vi "Cipher to Number.vi"(8 "error in (no error)":errorcluster, 11 "Cipers":i32[](array[numeric])) -> (0 "error out":errorcluster, 1 "Negative":bool, 3 "Number":i32)   [LabVIEW 2018, in "Resistance Values.lvlib"]
uses:
  Resistance Values.lvlib
  <vilib>/Utility/error.llb/Error Cluster From Error Code.vi
  <vilib>/ErrorRing/Error Ring.xnode
panel:
  # "index = 0 ->LDS"
  # "index = 1 ->......"
  # "index = n -> MDS"
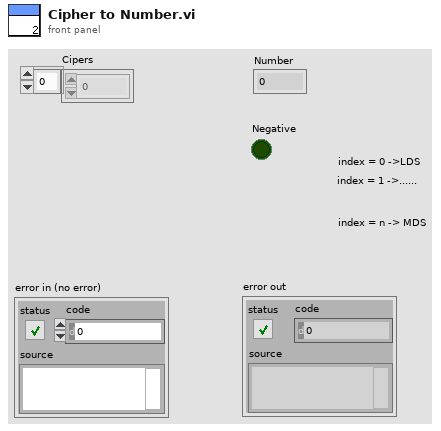
[diagram p1: front panel]
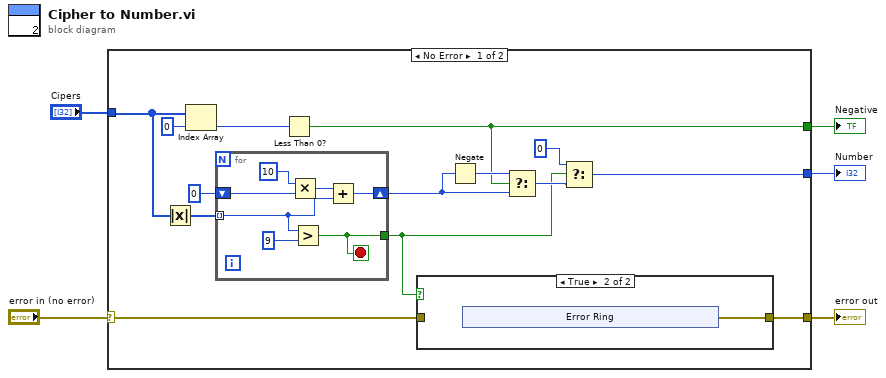
[diagram p0: block diagram]
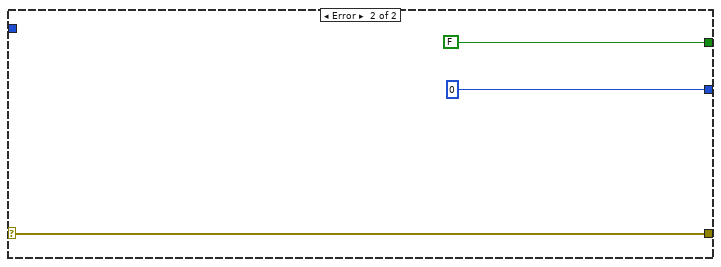
[diagram p3: hidden frame]
diagram:
  n1 = case shown="No Error" "error in (no error)" {
    selector: "error in (no error)" -> [w8 w36]
    tunnel: "Cipers" -> [w16 _]
    tunnel: [w13 FALSE] -> w3
    tunnel: [w9 0] -> w2
    tunnel: [w6 w36] -> w1
    frame No Error {
      n2 = Absolute Value(x=w16) -> (abs(x)=w17:i32[])
      n3 = Index Array(array=w16, index=0) -> (element=w18:i32)
      n4 = for {
        tunnel: w17 -> [w29] mode=indexing
        shift-right: [w30] -> w12
        shift-left: 0 -> [w33]
        tunnel: [w27] -> w7
        stop <- w27 stop-if-true
        n5 = Multiply(x=10, y=w33) -> (x*y=w31:i32)
        n6 = Greater?(x=w29, y=9) -> (0:w27:bool)
        n7 = Add(x=w31, y=w29) -> (x+y=w30:i32)
      }
      n8 = Less Than 0?(x=w18) -> (x < 0?=w13:bool)
      n9 = case shown="True" w7 {
        tunnel: w8 -> [w20 _]
        tunnel: [w20 w21] -> w6
        frame False {
        }
        frame True {
          n10 = xnode "Error Ring"() -> ("error out"=w21:errorcluster)
        }
      }
      n11 = Negate(x=w12) -> (-x=w14:i32)
      n12 = Select(t=w14, s=w13, f=w12) -> (s? t:f=w11:i32)
      n13 = Select(t=0, s=w7, f=w11) -> (s? t:f=w9:i32)
    }
    frame Error {
    }
  }
  "Number" <- w2
  "Negative" <- w3
  "error out" <- w1
